vi "Build Path if Relative.vi"(1 "Relative or Absolute Path":path, 2 "Base Path":path) -> (0 "Path Out":path)   [LabVIEW 2016, in "SLL File IO.lvlib"]
doc: "Builds base path with incoming path, if the incoming path is relative. If absolute, it returns the incoming path as such. \n\nThis VI would be useful to allow users to provide either relative paths or absolute paths as input and this VI takes care of converting them to the absolute paths."
uses:
  SLL File IO.lvlib
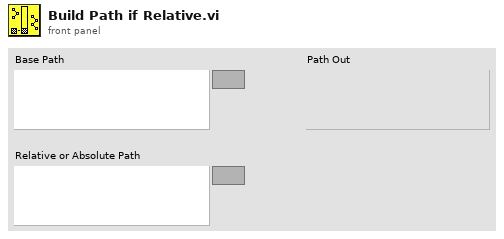
[diagram p1: front panel]
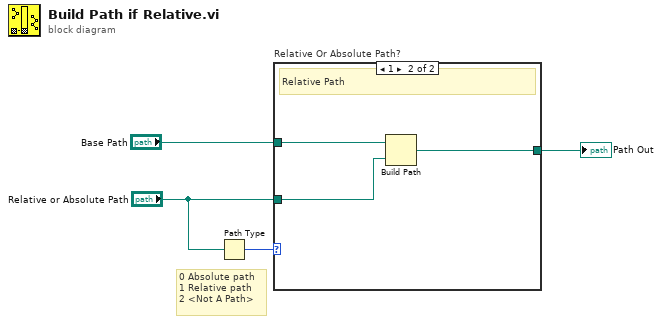
[diagram p0: block diagram]
diagram:
  # "0 Absolute path \n1 Relative path \n2 <Not A Path>"
  n1 = Path Type(1:"Relative or Absolute Path") -> (0:w4:i16)
  n2 = case "Relative Or Absolute Path?" shown="1" w4 {
    tunnel: "Base Path" -> [_ w8]
    tunnel: "Relative or Absolute Path" -> [w5 w7]
    tunnel: [w5 w6] -> w1
    frame 0, Default {
      # "Absolute or Not a Path. \nDon't Build"
    }
    frame 1 {
      # "Relative Path"
      n3 = Build Path(base path=w8, name or relative path=w7) -> (appended path=w6:path)
    }
  }
  "Path Out" <- w1
